vi "nanocal -- nuclear schottky fit V7.vi"() -> ()   [LabVIEW 2021] (continued)
\"T\" -> 0.830000000000   ,  \"B\" -> 0.000000000000   ,  \"θ\" -> 0.000000000000   ,  \"Reoff\" -> -3028571.428571429100   ,  \"Imoff\" -> 0.000000000000   ,  \"στ1\" -> 0.003777268036   ,  \"στS\" -> 0.001674973783   ,  \"στN\" -> 0.000298996570    |>   , \n\"IDS0417_220525_RAW_cal__sam_\" ->   <|    \"ζ\" -> 0.020422056832   ,  \"τ1\" -> 0.006457484957   ,  \"τS\" -> 0.019722165301   ,  \"τN\" -> 0.000729413719   ,  \"τC\" -> 0.001622930071   ,  \"κ0\" -> 0.000000005380   ,  \"mm1\" -> 0.000030097695   ,  \"mm2\" -> 0.006162713408   ,  \"mm3\" -> 0.022756846254   ,  \"T\" -> 0.830000000000   ,  \"B\" -> 0.000000000000   ,  \"θ\" -> 0.000000000000   ,  \"Reoff\" -> -2081632.653061224150   ,  \"Imoff\" -> 0.000000000000   ,  \"στ1\" -> 0.000977899540   ,  \"στS\" -> 0.002370947727   ,  \"στN\" -> 0.000160479256    |>   , \n\"IDS0418_220525_RAW_cal__ref_\" ->   <|    \"ζ\" -> 0.022904137166   ,  \"τ1\" -> 0.004842430213   ,  \"τS\" -> 0.021231337399   ,  \"τN\" -> 0.000595878691   ,  \"τC\" -> 0.001701256533   ,  \"κ0\" -> 0.000000006850   ,  \"mm1\" -> 0.000035378969   ,  \"mm2\" -> 0.004689611444   ,  \"mm3\" -> 0.024145845974   ,  \"T\" -> 1.120000000000   ,  \"B\" -> 0.000000000000   ,  \"θ\" -> 0.000000000000   ,  \"Reoff\" -> -1314285.714285716420   ,  \"Imoff\" -> 0.000000000000   ,  \"στ1\" -> 0.000594455147   ,  \"στS\" -> 0.001847173468   ,  \"στN\" -> 0.000101337306    |>   , \n\"IDS0418_220525_RAW_cal__sam_\" ->   <|    \"ζ\" -> 0.010833914814   ,  \"τ1\" -> 0.006105280968   ,  \"τS\" -> 0.027771405990   ,  \"τN\" -> 0.000655710517   ,  \"τC\" -> 0.001898693697   ,  \"κ0\" -> 0.000000007420   ,  \"mm1\" -> 0.000019072683   ,  \"mm2\" -> 0.005941306089   ,  \"mm3\" -> 0.030778689359   ,  \"T\" -> 1.120000000000   ,  \"B\" -> 0.000000000000   ,  \"θ\" -> 0.000000000000   ,  \"Reoff\" -> -608163.265306122367   ,  \"Imoff\" -> 0.000000000000   ,  \"στ1\" -> 0.001326459237   ,  \"στS\" -> 0.003728359065   ,  \"στN\" -> 0.000181682896    |>   , \n\"IDS0419_220525_RAW_cal__ref_\" ->   <|    \"ζ\" -> 0.019588015905   ,  \"τ1\" -> 0.004781626559   ,  \"τS\" -> 0.047742438651   ,  \"τN\" -> 0.000600848305   ,  \"τC\" -> 0.002316865749   ,  \"κ0\" -> 0.000000012200   ,  \"mm1\" -> 0.000042523875   ,  \"mm2\" -> 0.004719121437   ,  \"mm3\" -> 0.051627083026   ,  \"T\" -> 1.900000000000   ,  \"B\" -> 0.000000000000   ,  \"θ\" -> 0.000000000000   ,  \"Reoff\" -> -714285.714285716413   ,  \"Imoff\" -> 0.000000000000   ,  \"στ1\" -> 0.001059318885   ,  \"στS\" -> 0.005613918235   ,  \"στN\" -> 0.000174681152    |>   , \n\"IDS0419_220525_RAW_cal__sam_\" ->   <|    \"ζ\" -> 0.011595776290   ,  \"τ1\" -> 0.006117918264   ,  \"τS\" -> 0.061916055974   ,  \"τN\" -> 0.000669101537   ,  \"τC\" -> 0.002022450323   ,  \"κ0\" -> 0.000000012950   ,  \"mm1\" -> 0.000022465670   ,  \"mm2\" -> 0.006048051710   ,  \"mm3\" -> 0.065380732203   ,  \"T\" -> 1.900000000000   ,  \"B\" -> 0.000000000000   ,  \"θ\" -> 0.000000000000   ,  \"Reoff\" -> -608163.265306122367   ,  \"Imoff\" -> 0.000000000000   ,  \"στ1\" -> 0.001547930555   ,  \"στS\" -> 0.007827805463   ,  \"στN\" -> 0.000227173092    |>   , \n\"IDS0420_220525_RAW_cal__ref_\" ->   <|    \"ζ\" -> 0.020834428044   ,  \"τ1\" -> 0.004699063518   ,  \"τS\" -> 0.052089260804   ,  \"τN\" -> 0.000594934592   ,  \"τC\" -> 0.002174562230   ,  \"κ0\" -> 0.000000013800   ,  \"mm1\" -> 0.000042670178   ,  \"mm2\" -> 0.004643420551   ,  \"mm3\" -> 0.055969375493   ,  \"T\" -> 2.100000000000   ,  \"B\" -> 0.000000000000   ,  \"θ\" -> 0.000000000000   ,  \"Reoff\" -> -714285.714285716413   ,  \"Imoff\" -> 0.000000000000   ,  \"στ1\" -> 0.001320131062   ,  \"στS\" -> 0.004774189877   ,  \"στN\" -> 0.000170930701    |>   , \n\"IDS0420_220525_RAW_cal__sam_\" ->   <|    \"ζ\" -> 0.011850996022   ,  \"τ1\" -> 0.005764384736   ,  \"τS\" -> 0.066220067505   ,  \"τN\" -> 0.000645440877   ,  \"τC\" -> 0.002901198812   ,  \"κ0\" -> 0.000000014700   ,  \"mm1\" -> 0.000032584327   ,  \"mm2\" -> 0.005706320364   ,  \"mm3\" -> 0.070584610113   ,  \"T\" -> 2.100000000000   ,  \"B\" -> 0.000000000000   ,  \"θ\" -> 0.000000000000   ,  \"Reoff\" -> -461224.489795918343   ,  \"Imoff\" -> 0.000000000000   ,  \"στ1\" -> 0.000879947943   ,  \"στS\" -> 0.005816006372   ,  \"στN\" -> 0.000150645668    |>   , \n\"IDS0421_220525_RAW_cal__ref_\" ->   <|    \"ζ\" -> 0.022335092396   ,  \"τ1\" -> 0.004357676744   ,  \"τS\" -> 0.014734142286   ,  \"τN\" -> 0.000494755663   ,  \"τC\" -> 0.002291218216   ,  \"κ0\" -> 0.000000015200   ,  \"mm1\" -> 0.000043555244   ,  \"mm2\" -> 0.004196096690   ,  \"mm3\" -> 0.017978279817   ,  \"T\" -> 2.300000000000   ,  \"B\" -> 0.000000000000   ,  \"θ\" -> 0.000000000000   ,  \"Reoff\" -> -714285.714285716413   ,  \"Imoff\" -> 0.000000000000   ,  \"στ1\" -> 0.001017327919   ,  \"στS\" -> 0.002314643379   ,  \"στN\" -> 0.000146182526    |>   , \n\"IDS0421_220525_RAW_cal__sam_\" ->   <|    \"ζ\" -> 0.017472306497   ,  \"τ1\" -> 0.005884707777   ,  \"τS\" -> 0.018273540555   ,  \"τN\" -> 0.000393530305   ,  \"τC\" -> 0.002873982576   ,  \"κ0\" -> 0.000000016000   ,  \"mm1\" -> 0.000042829990   ,  \"mm2\" -> 0.005738391469   ,  \"mm3\" -> 0.021970696537   ,  \"T\" -> 2.300000000000   ,  \"B\" -> 0.000000000000   ,  \"θ\" -> 0.000000000000   ,  \"Reoff\" -> -616326.530612244968   ,  \"Imoff\" -> 0.000000000000   ,  \"στ1\" -> 0.001449504442   ,  \"στS\" -> 0.003094967894   ,  \"στN\" -> 0.000132016087    |>   , \n\"IDS0422_220525_RAW_cal__ref_\" ->   <|    \"ζ\" -> 0.018555902016   ,  \"τ1\" -> 0.004075291246   ,  \"τS\" -> 0.009145270052   ,  \"τN\" -> 0.000208864759   ,  \"τC\" -> 0.002022167505   ,  \"κ0\" -> 0.000000022500   ,  \"mm1\" -> 0.000030348931   ,  \"mm2\" -> 0.003960776557   ,  \"mm3\" -> 0.011634042483   ,  \"T\" -> 3.100000000000   ,  \"B\" -> 0.000000000000   ,  \"θ\" -> 0.000000000000   ,  \"Reoff\" -> -371428.571428570896   ,  \"Imoff\" -> 0.000000000000   ,  \"στ1\" -> 0.000657121780   ,  \"στS\" -> 0.001216403398   ,  \"στN\" -> 0.000050486757    |>   , \n\"IDS0422_220525_RAW_cal__sam_\" ->   <|    \"ζ\" -> 0.013782660001   ,  \"τ1\" -> 0.005602489845   ,  \"τS\" -> 0.011122141420   ,  \"τN\" -> 0.000341635093   ,  \"τC\" -> 0.002887063483   ,  \"κ0\" -> 0.000000023500   ,  \"mm1\" -> 0.000031317292   ,  \"mm2\" -> 0.005389288482   ,  \"mm3\" -> 0.014690725401   ,  \"T\" -> 3.100000000000   ,  \"B\" -> 0.000000000000   ,  \"θ\" -> 0.000000000000   ,  \"Reoff\" -> -338775.510204081656   ,  \"Imoff\" -> 0.000000000000   ,  \"στ1\" -> 0.000787586702   ,  \"στS\" -> 0.001319427978   ,  \"στN\" -> 0.000072408344    |>   , \n\"IDS0424_220526_RAW_cal__ref_\" ->   <|    \"ζ\" -> 0.257865003377   ,  \"τ1\" -> 0.052975439100   ,  \"τS\" -> 0.072879585760   ,  \"τN\" -> 0.046129702285   ,  \"τC\" -> 0.000850997737   ,  \"κ0\" -> 0.000000000770   ,  \"mm1\" -> 0.000173173247   ,  \"mm2\" -> 0.027881728109   ,  \"mm3\" -> 0.175469153990   ,  \"T\" -> 0.190000000000   ,  \"B\" -> 10.000000000000   ,  \"θ\" -> 0.000000000000   ,  \"Reoff\" -> -49000000.000000000000   ,  \"Imoff\" -> 0.000000000000   ,  \"στ1\" -> 0.038419382366   ,  \"στS\" -> 0.010252018344   ,  \"στN\" -> 0.015460977129    |>   , \n\"IDS0424_220526_RAW_cal__sam_\" ->   <|    \"ζ\" -> 0.143096873941   ,  \"τ1\" -> 0.119527741552   ,  \"τS\" -> 0.213771204505   ,  \"τN\" -> 0.133065206622   ,  \"τC\" -> 0.001041786526   ,  \"κ0\" -> 0.000000000890   ,  \"mm1\" -> 0.000129929317   ,  \"mm2\" -> 0.064852834373   ,  \"mm3\" -> 0.452054381716   ,  \"T\" -> 0.190000000000   ,  \"B\" -> 10.000000000000   ,  \"θ\" -> 0.000000000000   ,  \"Reoff\" -> -41461224.489795915800   ,  \"Imoff\" -> 0.000000000000   ,  \"στ1\" -> 0.142328196867   ,  \"στS\" -> 0.153709890516   ,  \"στN\" -> 0.034979737706    |>   , \n\"IDS0425_220526_RAW_cal__ref_\" ->   <|    \"ζ\" -> 0.150640974704   ,  \"τ1\" -> 0.034197272609   ,  \"τS\" -> 0.049670713863   ,  \"τN\" -> 0.019296596370   ,  \"τC\" -> 0.000986151726   ,  \"κ0\" -> 0.000000001118   ,  \"mm1\" -> 0.000127191823   ,  \"mm2\" -> 0.021308290346   ,  \"mm3\" -> 0.093104555235   ,  \"T\" -> 0.250000000000   ,  \"B\" -> 10.000000000000   ,  \"θ\" -> 0.000000000000   ,  \"Reoff\" -> -20330612.244897961600   ,  \"Imoff\" -> 0.000000000000   ,  \"στ1\" -> 0.016426599332   ,  \"στS\" -> 0.002938321228   ,  \"στN\" -> 0.003825151273    |>   , \n\"IDS0425_220526_RAW_cal__sam_\" ->   <|    \"ζ\" -> 0.080613368975   ,  \"τ1\" -> 0.039981630615   ,  \"τS\" -> 0.067451052819   ,  \"τN\" -> 0.024952731947   ,  \"τC\" -> 0.001301901326   ,  \"κ0\" -> 0.000000001270   ,  \"mm1\" -> 0.000095538727   ,  \"mm2\" -> 0.025680137218   ,  \"mm3\" -> 0.115360621158   ,  \"T\" -> 0.250000000000   ,  \"B\" -> 10.000000000000   ,  \"θ\" -> 0.000000000000   ,  \"Reoff\" -> -15077551.020408168400   ,  \"Imoff\" -> 0.000000000000   ,  \"στ1\" -> 0.017921325903   ,  \"στS\" -> 0.008554959302   ,  \"στN\" -> 0.012696106226    |>   , \n\"IDS0426_220526_RAW_cal__ref_\" ->   <|    \"ζ\" -> 0.110651122840   ,  \"τ1\" -> 0.023688979566   ,  \"τS\" -> 0.041888104291   ,  \"τN\" -> 0.009400965947   ,  \"τC\" -> 0.001054144270   ,  \"κ0\" -> 0.000000001430   ,  \"mm1\" -> 0.000102915193   ,  \"mm2\" -> 0.017560405745   ,  \"mm3\" -> 0.064044066348   ,  \"T\" -> 0.300000000000   ,  \"B\" -> 10.000000000000   ,  \"θ\" -> 0.000000000000   ,  \"Reoff\" -> -13408163.265306122600   ,  \"Imoff\" -> 0.000000000000   ,  \"στ1\" -> 0.009988334429   ,  \"στS\" -> 0.001537868285   ,  \"στN\" -> 0.001719296338    |>   , \n\"IDS0426_220526_RAW_cal__sam_\" ->   <|    \"ζ\" -> 0.000000000000   ,  \"τ1\" -> 0.000000000000   ,  \"τS\" -> 0.000000000000   ,  \"τN\" -> 0.000000000000   ,  \"τC\" -> 0.000000000000   ,  \"κ0\" -> 0.000000000000   ,  \"mm1\" -> 0.000000000000   ,  \"mm2\" -> 0.000000000000   ,  \"mm3\" -> 0.000000000000   ,  \"T\" -> 0.300000000000   ,  \"B\" -> 10.000000000000   ,  \"θ\" -> 0.000000000000   ,  \"Reoff\" -> 0.000000000000   ,  \"Imoff\" -> 0.000000000000   ,  \"στ1\" -> 0.000000000000   ,  \"στS\" -> 0.000000000000   ,  \"στN\" -> 0.000000000000    |>   , \n\"IDS0427_220526_RAW_cal__ref_\" ->   <|    \"ζ\" -> 0.400378368532   ,  \"τ1\" -> 0.070020543839   ,  \"τS\" -> 0.131128875469   ,  \"τN\" -> 0.110503953528   ,  \"τC\" -> 0.000929381263   ,  \"κ0\" -> 0.000000000547   ,  \"mm1\" -> 0.000264755544   ,  \"mm2\" -> 0.034447529222   ,  \"mm3\" -> 0.374615027191   ,  \"T\" -> 0.150000000000   ,  \"B\" -> 10.000000000000   ,  \"θ\" -> 0.000000000000   ,  \"Reoff\" -> -90065306.122448980800   ,  \"Imoff\" -> 0.000000000000   ,  \"στ1\" -> 0.115545840550   ,  \"στS\" -> 0.062145974598   ,  \"στN\" -> 0.087083233243    |>   , \n\"IDS0427_220526_RAW_cal__sam_\" ->   <|    \"ζ\" -> 0.000000000000   ,  \"τ1\" -> 0.000000000000   ,  \"τS\" -> 0.000000000000   ,  \"τN\" -> 0.000000000000   ,  \"τC\" -> 0.000000000000   ,  \"κ0\" -> 0.000000000000   ,  \"mm1\" -> 0.000000000000   ,  \"mm2\" -> 0.000000000000   ,  \"mm3\" -> 0.000000000000   ,  \"T\" -> 0.150000000000   ,  \"B\" -> 10.000000000000   ,  \"θ\" -> 0.000000000000   ,  \"Reoff\" -> 0.000000000000   ,  \"Imoff\" -> 0.000000000000   ,  \"στ1\" -> 0.000000000000   ,  \"στS\" -> 0.000000000000   ,  \"στN\" -> 0.000000000000    |>   , \n\"IDS0428_220526_RAW_cal__ref_\" ->   <|    \"ζ\" -> 0.082438962756   ,  \"τ1\" -> 0.024345135189   ,  \"τS\" -> 0.039010983719   ,  \"τN\" -> 0.005604008996   ,  \"τC\" -> 0.001011795266   ,  \"κ0\" -> 0.000000001850   ,  \"mm1\" -> 0.000075386231   ,  \"mm2\" -> 0.019395489677   ,  \"mm3\" -> 0.054179060985   ,  \"T\" -> 0.360000000000   ,  \"B\" -> 10.000000000000   ,  \"θ\" -> 0.000000000000   ,  \"Reoff\" -> -9632653.061224490410   ,  \"Imoff\" -> 0.000000000000   ,  \"στ1\" -> 0.001903743103   ,  \"στS\" -> 0.000574153374   ,  \"στN\" -> 0.002568840036    |>   , \n\"IDS0428_220526_RAW_cal__sam_\" ->   <|    \"ζ\" -> 0.000000000000   ,  \"τ1\" -> 0.000000000000   ,  \"τS\" -> 0.000000000000   ,  \"τN\" -> 0.000000000000   ,  \"τC\" -> 0.000000000000   ,  \"κ0\" -> 0.000000000000   ,  \"mm1\" -> 0.000000000000   ,  \"mm2\" -> 0.000000000000   ,  \"mm3\" -> 0.000000000000   ,  \"T\" -> 0.360000000000   ,  \"B\" -> 10.000000000000   ,  \"θ\" -> 0.000000000000   ,  \"Reoff\" -> 0.000000000000   ,  \"Imoff\" -> 0.000000000000   ,  \"στ1\" -> 0.000000000000   ,  \"στS\" -> 0.000000000000   ,  \"στN\" -> 0.000000000000    |>   , \n\"IDS0429_220526_RAW_cal__ref_\" ->   <|    \"ζ\" -> 0.070312011413   ,  \"τ1\" -> 0.022685637424   ,  \"τS\" -> 0.038017817435   ,  \"τN\" -> 0.003686111033   ,  \"τC\" -> 0.000858092615   ,  \"κ0\" -> 0.000000002230   ,  \"mm1\" -> 0.000055279779   ,  \"mm2\" -> 0.019266175315   ,  \"mm3\" -> 0.048858490507   ,  \"T\" -> 0.420000000000   ,  \"B\" -> 10.000000000000   ,  \"θ\" -> 0.000000000000   ,  \"Reoff\" -> -9632653.061224490410   ,  \"Imoff\" -> 0.000000000000   ,  \"στ1\" -> 0.001355990341   ,  \"στS\" -> 0.000271524957   ,  \"στN\" -> 0.000140246830    |>   , \n\"IDS0429_220526_RAW_cal__sam_\" ->   <|    \"ζ\" -> 0.000000000000   ,  \"τ1\" -> 0.000000000000   ,  \"τS\" -> 0.000000000000   ,  \"τN\" -> 0.000000000000   ,  \"τC\" -> 0.000000000000   ,  \"κ0\" -> 0.000000000000   ,  \"mm1\" -> 0.000000000000   ,  \"mm2\" -> 0.000000000000   ,  \"mm3\" -> 0.000000000000   ,  \"T\" -> 0.420000000000   ,  \"B\" -> 10.000000000000   ,  \"θ\" -> 0.000000000000   ,  \"Reoff\" -> 0.000000000000   ,  \"Imoff\" -> 0.000000000000   ,  \"στ1\" -> 0.000000000000   ,  \"στS\" -> 0.000000000000   ,  \"στN\" -> 0.000000000000    |>   , \n\"IDS0430_220526_RAW_cal__ref_\" ->   <|    \"ζ\" -> 0.045461152604   ,  \"τ1\" -> 0.022205538452   ,  \"τS\" -> 0.038393095410   ,  \"τN\" -> 0.002129809404   ,  \"τC\" -> 0.001500655488   ,  \"κ0\" -> 0.000000002910   ,  \"mm1\" -> 0.000062998174   ,  \"mm2\" -> 0.020118168551   ,  \"mm3\" -> 0.045890149989   ,  \"T\" -> 0.520000000000   ,  \"B\" -> 10.000000000000   ,  \"θ\" -> 0.000000000000   ,  \"Reoff\" -> -3224489.795918375260   ,  \"Imoff\" -> 0.000000000000   ,  \"στ1\" -> 0.001544196925   ,  \"στS\" -> 0.000197668706   ,  \"στN\" -> 0.000070756968    |>   , \n\"IDS0430_220526_RAW_cal__sam_\" ->   <|    \"ζ\" -> 0.000000000000   ,  \"τ1\" -> 0.000000000000   ,  \"τS\" -> 0.000000000000   ,  \"τN\" -> 0.000000000000   ,  \"τC\" -> 0.000000000000   ,  \"κ0\" -> 0.000000000000   ,  \"mm1\" -> 0.000000000000   ,  \"mm2\" -> 0.000000000000   ,  \"mm3\" -> 0.000000000000   ,  \"T\" -> 0.520000000000   ,  \"B\" -> 10.000000000000   ,  \"θ\" -> 0.000000000000   ,  \"Reoff\" -> 0.000000000000   ,  \"Imoff\" -> 0.000000000000   ,  \"στ1\" -> 0.000000000000   ,  \"στS\" -> 0.000000000000   ,  \"στN\" -> 0.000000000000    |>   , \n\"IDS0431_220527_RAW_cal__ref_\" ->   <|    \"ζ\" -> 0.560959524386   ,  \"τ1\" -> 0.162135875123   ,  \"τS\" -> 0.311559023690   ,  \"τN\" -> 0.235565493895   ,  \"τC\" -> 0.000943331482   ,  \"κ0\" -> 0.000000000415   ,  \"mm1\" -> 0.000338581832   ,  \"mm2\" -> 0.084703245290   ,  \"mm3\" -> 0.932076606233   ,  \"T\" -> 0.120000000000   ,  \"B\" -> 10.000000000000   ,  \"θ\" -> 0.000000000000   ,  \"Reoff\" -> -130387755.102040812000   ,  \"Imoff\" -> 0.000000000000   ,  \"στ1\" -> 0.196821258023   ,  \"στS\" -> 0.124985342591   ,  \"στN\" -> 0.122755892139    |>   , \n\"IDS0431_220527_RAW_cal__sam_\" ->   <|    \"ζ\" -> 0.000000000000   ,  \"τ1\" -> 0.000000000000   ,  \"τS\" -> 0.000000000000   ,  \"τN\" -> 0.000000000000   ,  \"τC\" -> 0.000000000000   ,  \"κ0\" -> 0.000000000000   ,  \"mm1\" -> 0.000000000000   ,  \"mm2\" -> 0.000000000000   ,  \"mm3\" -> 0.000000000000   ,  \"T\" -> 0.120000000000   ,  \"B\" -> 10.000000000000   ,  \"θ\" -> 0.000000000000   ,  \"Reoff\" -> 0.000000000000   ,  \"Imoff\" -> 0.000000000000   ,  \"στ1\" -> 0.000000000000   ,  \"στS\" -> 0.000000000000   ,  \"στN\" -> 0.000000000000    |>   , \n\"IDS0432_220527_RAW_cal__ref_\" ->   <|    \"ζ\" -> 0.302881771202   ,  \"τ1\" -> 0.053970650610   ,  \"τS\" -> 0.084832458604   ,  \"τN\" -> 0.070036651320   ,  \"τC\" -> 0.000864371133   ,  \"κ0\" -> 0.000000000675   ,  \"mm1\" -> 0.000199736141   ,  \"mm2\" -> 0.026051282095   ,  \"mm3\" -> 0.230360143749   ,  \"T\" -> 0.170000000000   ,  \"B\" -> 10.000000000000   ,  \"θ\" -> 0.000000000000   ,  \"Reoff\" -> -65714285.714285716400   ,  \"Imoff\" -> 0.000000000000   ,  \"στ1\" -> 0.042116863127   ,  \"στS\" -> 0.016985307293   ,  \"στN\" -> 0.023565277591    |>   , \n\"IDS0432_220527_RAW_cal__sam_\" ->   <|    \"ζ\" -> 0.000000000000   ,  \"τ1\" -> 0.000000000000   ,  \"τS\" -> 0.000000000000   ,  \"τN\" -> 0.000000000000   ,  \"τC\" -> 0.000000000000   ,  \"κ0\" -> 0.000000000000   ,  \"mm1\" -> 0.000000000000   ,  \"mm2\" -> 0.000000000000   ,  \"mm3\" -> 0.000000000000   ,  \"T\" -> 0.170000000000   ,  \"B\" -> 10.000000000000   ,  \"θ\" -> 0.000000000000   ,  \"Reoff\" -> 0.000000000000   ,  \"Imoff\" -> 0.000000000000   ,  \"στ1\" -> 0.000000000000   ,  \"στS\" -> 0.000000000000   ,  \"στN\" -> 0.000000000000    |>   , \n\"IDS0433_220527_RAW_cal__ref_\" ->   <|    \"ζ\" -> 0.035999178559   ,  \"τ1\" -> 0.021236822586   ,  \"τS\" -> 0.040779763241   ,  \"τN\" -> 0.001074221992   ,  \"τC\" -> 0.001739718615   ,  \"κ0\" -> 0.000000003576   ,  \"mm1\" -> 0.000058137989   ,  \"mm2\" -> 0.020282386509   ,  \"mm3\" -> 0.045996711024   ,  \"T\" -> 0.620000000000   ,  \"B\" -> 10.000000000000   ,  \"θ\" -> 0.000000000000   ,  \"Reoff\" -> -1959183.673469394450   ,  \"Imoff\" -> 0.000000000000   ,  \"στ1\" -> 0.001449693425   ,  \"στS\" -> 0.000173563135   ,  \"στN\" -> 0.000045450535    |>   , \n\"IDS0433_220527_RAW_cal__sam_\" ->   <|    \"ζ\" -> 0.000000000000   ,  \"τ1\" -> 0.000000000000   ,  \"τS\" -> 0.000000000000   ,  \"τN\" -> 0.000000000000   ,  \"τC\" -> 0.000000000000   ,  \"κ0\" -> 0.000000000000   ,  \"mm1\" -> 0.000000000000   ,  \"mm2\" -> 0.000000000000   ,  \"mm3\" -> 0.000000000000   ,  \"T\" -> 0.620000000000   ,  \"B\" -> 10.000000000000   ,  \"θ\" -> 0.000000000000   ,  \"Reoff\" -> 0.000000000000   ,  \"Imoff\" -> 0.000000000000   ,  \"στ1\" -> 0.000000000000   ,  \"στS\" -> 0.000000000000   ,  \"στN\" -> 0.000000000000    |>   , \n\"IDS0434_220527_RAW_cal__ref_\" ->   <|    \"ζ\" -> 0.027519355554   ,  \"τ1\" -> 0.020590521074   ,  \"τS\" -> 0.048137141101   ,  \"τN\" -> 0.000693113139   ,  \"τC\" -> 0.001789335146   ,  \"κ0\" -> 0.000000004950   ,  \"mm1\" -> 0.000046291190   ,  \"mm2\" -> 0.020129239579   ,  \"mm3\" -> 0.052378356819   ,  \"T\" -> 0.820000000000   ,  \"B\" -> 10.000000000000   ,  \"θ\" -> 0.000000000000   ,  \"Reoff\" -> -1326530.612244904040   ,  \"Imoff\" -> 0.000000000000   ,  \"στ1\" -> 0.000620759114   ,  \"στS\" -> 0.000219619310   ,  \"στN\" -> 0.000010903062    |>   , \n\"IDS0434_220527_RAW_cal__sam_\" ->   <|    \"ζ\" -> 0.000000000000   ,  \"τ1\" -> 0.000000000000   ,  \"τS\" -> 0.000000000000   ,  \"τN\" -> 0.000000000000   ,  \"τC\" -> 0.000000000000   ,  \"κ0\" -> 0.000000000000   ,  \"mm1\" -> 0.000000000000   ,  \"mm2\" -> 0.000000000000   ,  \"mm3\" -> 0.000000000000   ,  \"T\" -> 0.820000000000   ,  \"B\" -> 10.000000000000   ,  \"θ\" -> 0.000000000000   ,  \"Reoff\" -> 0.000000000000   ,  \"Imoff\" -> 0.000000000000   ,  \"στ1\" -> 0.000000000000   ,  \"στS\" -> 0.000000000000   ,  \"στN\" -> 0.000000000000    |>   , \n\"IDS0435_220527_RAW_cal__ref_\" ->   <|    \"ζ\" -> 0.020842861739   ,  \"τ1\" -> 0.020135384195   ,  \"τS\" -> 0.018612634604   ,  \"τN\" -> 0.000305402785   ,  \"τC\" -> 0.002204389625   ,  \"κ0\" -> 0.000000007040   ,  \"mm1\" -> 0.000040405722   ,  \"mm2\" -> 0.018212466466   ,  \"mm3\" -> 0.023399245059   ,  \"T\" -> 1.120000000000   ,  \"B\" -> 10.000000000000   ,  \"θ\" -> 0.000000000000   ,  \"Reoff\" -> -693877.551020413636   ,  \"Imoff\" -> 0.000000000000   ,  \"στ1\" -> 0.001444867016   ,  \"στS\" -> 0.000117188914   ,  \"στN\" -> 0.000006503631    |>   , \n\"IDS0435_220527_RAW_cal__sam_\" ->   <|    \"ζ\" -> 0.000000000000   ,  \"τ1\" -> 0.000000000000   ,  \"τS\" -> 0.000000000000   ,  \"τN\" -> 0.000000000000   ,  \"τC\" -> 0.000000000000   ,  \"κ0\" -> 0.000000000000   ,  \"mm1\" -> 0.000000000000   ,  \"mm2\" -> 0.000000000000   ,  \"mm3\" -> 0.000000000000   ,  \"T\" -> 1.120000000000   ,  \"B\" -> 10.000000000000   ,  \"θ\" -> 0.000000000000   ,  \"Reoff\" -> 0.000000000000   ,  \"Imoff\" -> 0.000000000000   ,  \"στ1\" -> 0.000000000000   ,  \"στS\" -> 0.000000000000   ,  \"στN\" -> 0.000000000000    |>   , \n\"IDS0436_220527_RAW_cal__ref_\" ->   <|    \"ζ\" -> 0.020634042480   ,  \"τ1\" -> 0.020416898580   ,  \"τS\" -> 0.013006754143   ,  \"τN\" -> 0.000157221748   ,  \"τC\" -> 0.001868338850   ,  \"κ0\" -> 0.000000012250   ,  \"mm1\" -> 0.000033184482   ,  \"mm2\" -> 0.014698009084   ,  \"mm3\" -> 0.020989645793   ,  \"T\" -> 1.900000000000   ,  \"B\" -> 10.000000000000   ,  \"θ\" -> 0.000000000000   ,  \"Reoff\" -> -693877.551020413636   ,  \"Imoff\" -> 0.000000000000   ,  \"στ1\" -> 0.001009802597   ,  \"στS\" -> 0.000108538250   ,  \"στN\" -> 0.000005592624    |>   , \n\"IDS0436_220527_RAW_cal__sam_\" ->   <|    \"ζ\" -> 0.000000000000   ,  \"τ1\" -> 0.000000000000   ,  \"τS\" -> 0.000000000000   ,  \"τN\" -> 0.000000000000   ,  \"τC\" -> 0.000000000000   ,  \"κ0\" -> 0.000000000000   ,  \"mm1\" -> 0.000000000000   ,  \"mm2\" -> 0.000000000000   ,  \"mm3\" -> 0.000000000000   ,  \"T\" -> 1.900000000000   ,  \"B\" -> 10.000000000000   ,  \"θ\" -> 0.000000000000   ,  \"Reoff\" -> 0.000000000000   ,  \"Imoff\" -> 0.000000000000   ,  \"στ1\" -> 0.000000000000   ,  \"στS\" -> 0.000000000000   ,  \"στN\" -> 0.000000000000    |>   , \n\"IDS0437_220527_RAW_cal__ref_\" ->   <|    \"ζ\" -> 0.017700486500   ,  \"τ1\" -> 0.021195716861   ,  \"τS\" -> 0.009553240691   ,  \"τN\" -> 0.000096318625   ,  \"τC\" -> 0.001777778444   ,  \"κ0\" -> 0.000000022000   ,  \"mm1\" -> 0.000026199986   ,  \"mm2\" -> 0.011360732885   ,  \"mm3\" -> 0.021406923644   ,  \"T\" -> 3.100000000000   ,  \"B\" -> 10.000000000000   ,  \"θ\" -> 0.000000000000   ,  \"Reoff\" -> -326530.612244898453   ,  \"Imoff\" -> 0.000000000000   ,  \"στ1\" -> 0.003823035587   ,  \"στS\" -> 0.000080670014   ,  \"στN\" -> 0.000008312416    |>   , \n\"IDS0437_220527_RAW_cal__sam_\" ->   <|    \"ζ\" -> 0.000000000000   ,  \"τ1\" -> 0.000000000000   ,  \"τS\" -> 0.000000000000   ,  \"τN\" -> 0.000000000000   ,  \"τC\" -> 0.000000000000   ,  \"κ0\" -> 0.000000000000   ,  \"mm1\" -> 0.000000000000   ,  \"mm2\" -> 0.000000000000   ,  \"mm3\" -> 0.000000000000   ,  \"T\" -> 3.100000000000   ,  \"B\" -> 10.000000000000   ,  \"θ\" -> 0.000000000000   ,  \"Reoff\" -> 0.000000000000   ,  \"Imoff\" -> 0.000000000000   ,  \"στ1\" -> 0.000000000000   ,  \"στS\" -> 0.000000000000   ,  \"στN\" -> 0.000000000000    |>   , \n\"IDS0438_220527_RAW_cal__ref_\" ->   <|    \"ζ\" -> 0.017333863476   ,  \"τ1\" -> 0.021487771905   ,  \"τS\" -> 0.006060943357   ,  \"τN\" -> 0.000094743973   ,  \"τC\" -> 0.001680463551   ,  \"κ0\" -> 0.000000054800   ,  \"mm1\" -> 0.000022565233   ,  \"mm2\" -> 0.007769356044   ,  \"mm3\" -> 0.021638703353   ,  \"T\" -> 5.700000000000   ,  \"B\" -> 10.000000000000   ,  \"θ\" -> 0.000000000000   ,  \"Reoff\" -> -102040.816326530650   ,  \"Imoff\" -> 0.000000000000   ,  \"στ1\" -> 0.003634760564   ,  \"στS\" -> 0.000066823566   ,  \"στN\" -> 0.000004946508    |>   , \n\"IDS0438_220527_RAW_cal__sam_\" ->   <|    \"ζ\" -> 0.000000000000   ,  \"τ1\" -> 0.000000000000   ,  \"τS\" -> 0.000000000000   ,  \"τN\" -> 0.000000000000   ,  \"τC\" -> 0.000000000000   ,  \"κ0\" -> 0.000000000000   ,  \"mm1\" -> 0.000000000000   ,  \"mm2\" -> 0.000000000000   ,  \"mm3\" -> 0.000000000000   ,  \"T\" -> 5.700000000000   ,  \"B\" -> 10.000000000000   ,  \"θ\" -> 0.000000000000   ,  \"Reoff\" -> 0.000000000000   ,  \"Imoff\" -> 0.000000000000   ,  \"στ1\" -> 0.000000000000   ,  \"στS\" -> 0.000000000000   ,  \"στN\" -> 0.000000000000    |>   , \n\"IDS0439_220527_RAW_cal__ref_\" ->   <|    \"ζ\" -> 0.020515660719   ,  \"τ1\" -> 0.020182411708   ,  \"τS\" -> 0.016419895032   ,  \"τN\" -> 0.000240616919   ,  \"τC\" -> 0.002259910162   ,  \"κ0\" -> 0.000000008010   ,  \"mm1\" -> 0.000040116981   ,  \"mm2\" -> 0.017425178232   ,  \"mm3\" -> 0.021979340018   ,  \"T\" -> 1.280000000000   ,  \"B\" -> 10.000000000000   ,  \"θ\" -> 0.000000000000   ,  \"Reoff\" -> -693877.551020413636   ,  \"Imoff\" -> 0.000000000000   ,  \"στ1\" -> 0.001720696083   ,  \"στS\" -> 0.000105898596   ,  \"στN\" -> 0.000011441558    |>   , \n\"IDS0439_220527_RAW_cal__sam_\" ->   <|    \"ζ\" -> 0.000000000000   ,  \"τ1\" -> 0.000000000000   ,  \"τS\" -> 0.000000000000   ,  \"τN\" -> 0.000000000000   ,  \"τC\" -> 0.000000000000   ,  \"κ0\" -> 0.000000000000   ,  \"mm1\" -> 0.000000000000   ,  \"mm2\" -> 0.000000000000   ,  \"mm3\" -> 0.000000000000   ,  \"T\" -> 1.280000000000   ,  \"B\" -> 10.000000000000   ,  \"θ\" -> 0.000000000000   ,  \"Reoff\" -> 0.000000000000   ,  \"Imoff\" -> 0.000000000000   ,  \"στ1\" -> 0.000000000000   ,  \"στS\" -> 0.000000000000   ,  \"στN\" -> 0.000000000000    |>   , \n\"IDS0441_220527_RAW_cal__ref_\" ->   <|    \"ζ\" -> 0.245298177404   ,  \"τ1\" -> 0.085385227960   ,  \"τS\" -> 0.023089892303   ,  \"τN\" -> 0.011485885148   ,  \"τC\" -> 0.000787848696   ,  \"κ0\" -> 0.000000000810   ,  \"mm1\" -> 0.000151828666   ,  \"mm2\" -> 0.023847632864   ,  \"mm3\" -> 0.105230767769   ,  \"T\" -> 0.200000000000   ,  \"B\" -> 6.000000000000   ,  \"θ\" -> 0.000000000000   ,  \"Reoff\" -> -50367346.938775539400   ,  \"Imoff\" -> 0.000000000000   ,  \"στ1\" -> 0.073805144246   ,  \"στS\" -> 0.000832804395   ,  \"στN\" -> 0.007851231526    |>   , \n\"IDS0441_220527_RAW_cal__sam_\" ->   <|    \"ζ\" -> 0.000000000000   ,  \"τ1\" -> 0.000000000000   ,  \"τS\" -> 0.000000000000   ,  \"τN\" -> 0.000000000000   ,  \"τC\" -> 0.000000000000   ,  \"κ0\" -> 0.000000000000   ,  \"mm1\" -> 0.000000000000   ,  \"mm2\" -> 0.000000000000   ,  \"mm3\" -> 0.000000000000   ,  \"T\" -> 0.200000000000   ,  \"B\" -> 6.000000000000   ,  \"θ\" -> 0.000000000000   ,  \"Reoff\" -> 0.000000000000   ,  \"Imoff\" -> 0.000000000000   ,  \"στ1\" -> 0.000000000000   ,  \"στS\" -> 0.000000000000   ,  \"στN\" -> 0.000000000000    |>   , \n\"IDS0442_220528_RAW_cal__ref_\" ->   <|    \"ζ\" -> 0.649253803207   ,  \"τ1\" -> 0.189967266824   ,  \"τS\" -> 0.078891800944   ,  \"τN\" -> 0.111026532234   ,  \"τC\" -> 0.000810885423   ,  \"κ0\" -> 0.000000000435   ,  \"mm1\" -> 0.000318009867   ,  \"mm2\" -> 0.055339104870   ,  \"mm3\" -> 0.448344570802   ,  \"T\" -> 0.120000000000   ,  \"B\" -> 6.000000000000   ,  \"θ\" -> 0.000000000000   ,  \"Reoff\" -> -187755102.040816367000   ,  \"Imoff\" -> 0.000000000000   ,  \"στ1\" -> 0.116072095960   ,  \"στS\" -> 0.013830964310   ,  \"στN\" -> 0.055132667771    |>   , \n\"IDS0442_220528_RAW_cal__sam_\" ->   <|    \"ζ\" -> 0.000000000000   ,  \"τ1\" -> 0.000000000000   ,  \"τS\" -> 0.000000000000   ,  \"τN\" -> 0.000000000000   ,  \"τC\" -> 0.000000000000   ,  \"κ0\" -> 0.000000000000   ,  \"mm1\" -> 0.000000000000   ,  \"mm2\" -> 0.000000000000   ,  \"mm3\" -> 0.000000000000   ,  \"T\" -> 0.120000000000   ,  \"B\" -> 6.000000000000   ,  \"θ\" -> 0.000000000000   ,  \"Reoff\" -> 0.000000000000   ,  \"Imoff\" -> 0.000000000000   ,  \"στ1\" -> 0.000000000000   ,  \"στS\" -> 0.000000000000   ,  \"στN\" -> 0.000000000000    |>   , \n\"IDS0443_220528_RAW_cal__ref_\" ->   <|    \"ζ\" -> 0.445042406972   ,  \"τ1\" -> 0.128589504516   ,  \"τS\" -> 0.034654563108   ,  \"τN\" -> 0.043810211880   ,  \"τC\" -> 0.000810309510   ,  \"κ0\" -> 0.000000000605   ,  \"mm1\" -> 0.000246774346   ,  \"mm2\" -> 0.030747670130   ,  \"mm3\" -> 0.211790296861   ,  \"T\" -> 0.150000000000   ,  \"B\" -> 6.000000000000   ,  \"θ\" -> 0.000000000000   ,  \"Reoff\" -> -104489795.918367386000   ,  \"Imoff\" -> 0.000000000000   ,  \"στ1\" -> 0.161783937181   ,  \"στS\" -> 0.005303891089   ,  \"στN\" -> 0.043224722423    |>   , \n\"IDS0443_220528_RAW_cal__sam_\" ->   <|    \"ζ\" -> 0.000000000000   ,  \"τ1\" -> 0.000000000000   ,  \"τS\" -> 0.000000000000   ,  \"τN\" -> 0.000000000000   ,  \"τC\" -> 0.000000000000   ,  \"κ0\" -> 0.000000000000   ,  \"mm1\" -> 0.000000000000   ,  \"mm2\" -> 0.000000000000   ,  \"mm3\" -> 0.000000000000   ,  \"T\" -> 0.150000000000   ,  \"B\" -> 6.000000000000   ,  \"θ\" -> 0.000000000000   ,  \"Reoff\" -> 0.000000000000   ,  \"Imoff\" -> 0.000000000000   ,  \"στ1\" -> 0.000000000000   ,  \"στS\" -> 0.000000000000   ,  \"στN\" -> 0.000000000000    |>   , \n\"IDS0444_220528_RAW_cal__ref_\" ->   <|    \"ζ\" -> 0.346175274834   ,  \"τ1\" -> 0.111956082957   ,  \"τS\" -> 0.027343356843   ,  \"τN\" -> 0.025121384600   ,  \"τC\" -> 0.000749531065   ,  \"κ0\" -> 0.000000000740   ,  \"mm1\" -> 0.000189854194   ,  \"mm2\" -> 0.026751880765   ,  \"mm3\" -> 0.156390616794   ,  \"T\" -> 0.170000000000   ,  \"B\" -> 6.000000000000   ,  \"θ\" -> 0.000000000000   ,  \"Reoff\" -> -71183673.469387769700   ,  \"Imoff\" -> 0.000000000000   ,  \"στ1\" -> 0.050375037721   ,  \"στS\" -> 0.001079416051   ,  \"στN\" -> 0.009083705323    |>   , \n\"IDS0444_220528_RAW_cal__sam_\" ->   <|    \"ζ\" -> 0.000000000000   ,  \"τ1\" -> 0.000000000000   ,  \"τS\" -> 0.000000000000   ,  \"τN\" -> 0.000000000000   ,  \"τC\" -> 0.000000000000   ,  \"κ0\" -> 0.000000000000   ,  \"mm1\" -> 0.000000000000   ,  \"mm2\" -> 0.000000000000   ,  \"mm3\" -> 0.000000000000   ,  \"T\" -> 0.170000000000   ,  \"B\" -> 6.000000000000   ,  \"θ\" -> 0.000000000000   ,  \"Reoff\" -> 0.000000000000   ,  \"Imoff\" -> 0.000000000000   ,  \"στ1\" -> 0.000000000000   ,  \"στS\" -> 0.000000000000   ,  \"στN\" -> 0.000000000000    |>   , \n\"IDS0445_220528_RAW_cal__ref_\" ->   <|    \"ζ\" -> 0.167396769386   ,  \"τ1\" -> 0.076975995678   ,  \"τS\" -> 0.019126902976   ,  \"τN\" -> 0.005930151482   ,  \"τC\" -> 0.000960075113   ,  \"κ0\" -> 0.000000001240   ,  \"mm1\" -> 0.000132747039   ,  \"mm2\" -> 0.020623110398   ,  \"mm3\" -> 0.086431737778   ,  \"T\" -> 0.250000000000   ,  \"B\" -> 6.000000000000   ,  \"θ\" -> 0.000000000000   ,  \"Reoff\" -> -21224489.795918405100   ,  \"Imoff\" -> 0.000000000000   ,  \"στ1\" -> 0.058389287380   ,  \"στS\" -> 0.000426789295   ,  \"στN\" -> 0.003784929464    |>   , \n\"IDS0445_220528_RAW_cal__sam_\" ->   <|    \"ζ\" -> 0.000000000000   ,  \"τ1\" -> 0.000000000000   ,  \"τS\" -> 0.000000000000   ,  \"τN\" -> 0.000000000000   ,  \"τC\" -> 0.000000000000   ,  \"κ0\" -> 0.000000000000   ,  \"mm1\" -> 0.000000000000   ,  \"mm2\" -> 0.000000000000   ,  \"mm3\" -> 0.000000000000   ,  \"T\" -> 0.250000000000   ,  \"B\" -> 6.000000000000   ,  \"θ\" -> 0.000000000000   ,  \"Reoff\" -> 0.000000000000   ,  \"Imoff\" -> 0.000000000000   ,  \"στ1\" -> 0.000000000000   ,  \"στS\" -> 0.000000000000   ,  \"στN\" -> 0.000000000000    |>   , \n\"IDS0446_220528_RAW_cal__ref_\" ->   <|    \"ζ\" -> 0.116182318026   ,  \"τ1\" -> 0.081640310959   ,  \"τS\" -> 0.017704747394   ,  \"τN\" -> 0.003731217958   ,  \"τC\" -> 0.001140395347   ,  \"κ0\" -> 0.000000001560   ,  \"mm1\" -> 0.000112833833   ,  \"mm2\" -> 0.019484161721   ,  \"mm3\" -> 0.087110156248   ,  \"T\" -> 0.300000000000   ,  \"B\" -> 6.000000000000   ,  \"θ\" -> 0.000000000000   ,  \"Reoff\" -> -9836734.693877555430   ,  \"Imoff\" -> 0.000000000000   ,  \"στ1\" -> 0.008773282825   ,  \"στS\" -> 0.000191111466   ,  \"στN\" -> 0.000539753002    |>   , \n\"IDS0446_220528_RAW_cal__sam_\" ->   <|    \"ζ\" -> 0.000000000000   ,  \"τ1\" -> 0.000000000000   ,  \"τS\" -> 0.000000000000   ,  \"τN\" -> 0.000000000000   ,  \"τC\" -> 0.000000000000   ,  \"κ0\" -> 0.000000000000   ,  \"mm1\" -> 0.000000000000   ,  \"mm2\" -> 0.000000000000   ,  \"mm3\" -> 0.000000000000   ,  \"T\" -> 0.300000000000   ,  \"B\" -> 6.000000000000   ,  \"θ\" -> 0.000000000000   ,  \"Reoff\" -> 0.000000000000   ,  \"Imoff\" -> 0.000000000000   ,  \"στ1\" -> 0.000000000000   ,  \"στS\" -> 0.000000000000   ,  \"στN\" -> 0.000000000000    |>   , \n\"IDS0447_220528_RAW_cal__ref_\" ->   <|    \"ζ\" -> 0.082260507955   ,  \"τ1\" -> 0.097855412168   ,  \"τS\" -> 0.016892570352   ,  \"τN\" -> 0.002508450839   ,  \"τC\" -> 0.001377537548   ,  \"κ0\" -> 0.000000001980   ,  \"mm1\" -> 0.000097853534   ,  \"mm2\" -> 0.018911725587   ,  \"mm3\" -> 0.101220329644   ,  \"T\" -> 0.360000000000   ,  \"B\" -> 6.000000000000   ,  \"θ\" -> 0.000000000000   ,  \"Reoff\" -> -5918367.346938773990   ,  \"Imoff\" -> 0.000000000000   ,  \"στ1\" -> 0.011453835747   ,  \"στS\" -> 0.000169259584   ,  \"στN\" -> 0.000081203504    |>   , \n\"IDS0447_220528_RAW_cal__sam_\" ->   <|    \"ζ\" -> 0.000000000000   ,  \"τ1\" -> 0.000000000000   ,  \"τS\" -> 0.000000000000   ,  \"τN\" -> 0.000000000000   ,  \"τC\" -> 0.000000000000   ,  \"κ0\" -> 0.000000000000   ,  \"mm1\" -> 0.000000000000   ,  \"mm2\" -> 0.000000000000   ,  \"mm3\" -> 0.000000000000   ,  \"T\" -> 0.360000000000   ,  \"B\" -> 6.000000000000   ,  \"θ\" -> 0.000000000000   ,  \"Reoff\" -> 0.000000000000   ,  \"Imoff\" -> 0.000000000000   ,  \"στ1\" -> 0.000000000000   ,  \"στS\" -> 0.000000000000   ,  \"στN\" -> 0.000000000000    |>   , \n\"IDS0448_220528_RAW_cal__ref_\" ->   <|    \"ζ\" -> 0.062921401678   ,  \"τ1\" -> 0.104858235464   ,  \"τS\" -> 0.016995205436   ,  \"τN\" -> 0.001995569768   ,  \"τC\" -> 0.001676394953   ,  \"κ0\" -> 0.000000002390   ,  \"mm1\" -> 0.000091230686   ,  \"mm2\" -> 0.019175235813   ,  \"mm3\" -> 0.107453865317   ,  \"T\" -> 0.420000000000   ,  \"B\" -> 6.000000000000   ,  \"θ\" -> 0.000000000000   ,  \"Reoff\" -> -3224489.795918367800   ,  \"Imoff\" -> 0.000000000000   ,  \"στ1\" -> 0.006534185660   ,  \"στS\" -> 0.000117840372   ,  \"στN\" -> 0.000044604880    |>   , \n\"IDS0448_220528_RAW_cal__sam_\" ->   <|    \"ζ\" -> 0.000000000000   ,  \"τ1\" -> 0.000000000000   ,  \"τS\" -> 0.000000000000   ,  \"τN\" -> 0.000000000000   ,  \"τC\" -> 0.000000000000   ,  \"κ0\" -> 0.000000000000   ,  \"mm1\" -> 0.000000000000   ,  \"mm2\" -> 0.000000000000   ,  \"mm3\" -> 0.000000000000   ,  \"T\" -> 0.420000000000   ,  \"B\" -> 6.000000000000   ,  \"θ\" -> 0.000000000000   ,  \"Reoff\" -> 0.000000000000   ,  \"Imoff\" -> 0.000000000000   ,  \"στ1\" -> 0.000000000000   ,  \"στS\" -> 0.000000000000   ,  \"στN\" -> 0.000000000000    |>   , \n\"IDS0449_220528_RAW_cal__ref_\" ->   <|    \"ζ\" -> 0.047884623717   ,  \"τ1\" -> 0.131080457695   ,  \"τS\" -> 0.018007411450   ,  \"τN\" -> 0.000981367223   ,  \"τC\" -> 0.001725529599   ,  \"κ0\" -> 0.000000003050   ,  \"mm1\" -> 0.000072499299   ,  \"mm2\" -> 0.020333963628   ,  \"mm3\" -> 0.132297573561   ,  \"T\" -> 0.520000000000   ,  \"B\" -> 6.000000000000   ,  \"θ\" -> 0.000000000000   ,  \"Reoff\" -> -2734693.877551019190   ,  \"Imoff\" -> 0.000000000000   ,  \"στ1\" -> 0.004608574933   ,  \"στS\" -> 0.000117579650   ,  \"στN\" -> 0.000012752595    |>   , \n\"IDS0449_220528_RAW_cal__sam_\" ->   <|    \"ζ\" -> 0.000000000000   ,  \"τ1\" -> 0.000000000000   ,  \"τS\" -> 0.000000000000   ,  \"τN\" -> 0.000000000000   ,  \"τC\" -> 0.000000000000   ,  \"κ0\" -> 0.000000000000   ,  \"mm1\" -> 0.000000000000   ,  \"mm2\" -> 0.000000000000   ,  \"mm3\" -> 0.000000000000   ,  \"T\" -> 0.520000000000   ,  \"B\" -> 6.000000000000   ,  \"θ\" -> 0.000000000000   ,  \"Reoff\" -> 0.000000000000   ,  \"Imoff\" -> 0.000000000000   ,  \"στ1\" -> 0.000000000000   ,  \"στS\" -> 0.000000000000   ,  \"στN\" -> 0.000000000000    |>   , \n\"IDS0450_220528_RAW_cal__ref_\" ->   <|    \"ζ\" -> 0.039229464810   ,  \"τ1\" -> 0.132250871958   ,  \"τS\" -> 0.019567524350   ,  \"τN\" -> 0.000645572028   ,  \"τC\" -> 0.002216107396   ,  \"κ0\" -> 0.000000003710   ,  \"mm1\" -> 0.000075688104   ,  \"mm2\" -> 0.022339257593   ,  \"mm3\" -> 0.133058078988   ,  \"T\" -> 0.620000000000   ,  \"B\" -> 6.000000000000   ,  \"θ\" -> 0.000000000000   ,  \"Reoff\" -> -1836734.693877549840   ,  \"Imoff\" -> 0.000000000000   ,  \"στ1\" -> 0.013891983729   ,  \"στS\" -> 0.000275228505   ,  \"στN\" -> 0.000014669309    |>   , \n\"IDS0450_220528_RAW_cal__sam_\" ->   <|    \"ζ\" -> 0.000000000000   ,  \"τ1\" -> 0.000000000000   ,  \"τS\" -> 0.000000000000   ,  \"τN\" -> 0.000000000000   ,  \"τC\" -> 0.000000000000   ,  \"κ0\" -> 0.000000000000   ,  \"mm1\" -> 0.000000000000   ,  \"mm2\" -> 0.000000000000   ,  \"mm3\" -> 0.000000000000   ,  \"T\" -> 0.620000000000   ,  \"B\" -> 6.000000000000   ,  \"θ\" -> 0.000000000000   ,  \"Reoff\" -> 0.000000000000   ,  \"Imoff\" -> 0.000000000000   ,  \"στ1\" -> 0.000000000000   ,  \"στS\" -> 0.000000000000   ,  \"στN\" -> 0.000000000000    |>   , \n\"IDS0451_220528_RAW_cal__ref_\" ->   <|    \"ζ\" -> 0.026807399567   ,  \"τ1\" -> 0.154252177981   ,  \"τS\" -> 0.023590031432   ,  \"τN\" -> 0.000319958180   ,  \"τC\" -> 0.003023021175   ,  \"κ0\" -> 0.000000005180   ,  \"mm1\" -> 0.000070348215   ,  \"mm2\" -> 0.027105077142   ,  \"mm3\" -> 0.154650728056   ,  \"T\" -> 0.820000000000   ,  \"B\" -> 6.000000000000   ,  \"θ\" -> 0.000000000000   ,  \"Reoff\" -> -612244.897959182038   ,  \"Imoff\" -> 0.000000000000   ,  \"στ1\" -> 0.012428803494   ,  \"στS\" -> 0.000182806750   ,  \"στN\" -> 0.000002712737    |>   , \n\"IDS0451_220528_RAW_cal__sam_\" ->   <|    \"ζ\" -> 0.000000000000   ,  \"τ1\" -> 0.000000000000   ,  \"τS\" -> 0.000000000000   ,  \"τN\" -> 0.000000000000   ,  \"τC\" -> 0.000000000000   ,  \"κ0\" -> 0.000000000000   ,  \"mm1\" -> 0.000000000000   ,  \"mm2\" -> 0.000000000000   ,  \"mm3\" -> 0.000000000000   ,  \"T\" -> 0.820000000000   ,  \"B\" -> 6.000000000000   ,  \"θ\" -> 0.000000000000   ,  \"Reoff\" -> 0.000000000000   ,  \"Imoff\" -> 0.000000000000   ,  \"στ1\" -> 0.000000000000   ,  \"στS\" -> 0.000000000000   ,  \"στN\" -> 0.000000000000    |>   , \n\"IDS0452_220528_RAW_cal__ref_\" ->   <|    \"ζ\" -> 0.022314359927   ,  \"τ1\" -> 0.160926117275   ,  \"τS\" -> 0.032134640679   ,  \"τN\" -> 0.000145739971   ,  \"τC\" -> 0.002824145065   ,  \"κ0\" -> 0.000000007200   ,  \"mm1\" -> 0.000056854280   ,  \"mm2\" -> 0.035576714114   ,  \"mm3\" -> 0.161117390629   ,  \"T\" -> 1.120000000000   ,  \"B\" -> 6.000000000000   ,  \"θ\" -> 0.000000000000   ,  \"Reoff\" -> -702040.816326530649   ,  \"Imoff\" -> 0.000000000000   ,  \"στ1\" -> 0.054678579319   ,  \"στS\" -> 0.000310139427   ,  \"στN\" -> 0.000011071963    |>   , \n\"IDS0452_220528_RAW_cal__sam_\" ->   <|    \"ζ\" -> 0.000000000000   ,  \"τ1\" -> 0.000000000000   ,  \"τS\" -> 0.000000000000   ,  \"τN\" -> 0.000000000000   ,  \"τC\" -> 0.000000000000   ,  \"κ0\" -> 0.000000000000   ,  \"mm1\" -> 0.000000000000   ,  \"mm2\" -> 0.000000000000   ,  \"mm3\" -> 0.000000000000   ,  \"T\" -> 1.120000000000   ,  \"B\" -> 6.000000000000   ,  \"θ\" -> 0.000000000000   ,  \"Reoff\" -> 0.000000000000   ,  \"Imoff\" -> 0.000000000000   ,  \"στ1\" -> 0.000000000000   ,  \"στS\" -> 0.000000000000   ,  \"στN\" -> 0.000000000000    |>   , \n\"IDS0453_220529_RAW_cal__ref_\" ->   <|    \"ζ\" -> 0.018679261222   ,  \"τ1\" -> 0.150357444962   ,  \"τS\" -> 0.034780809519   ,  \"τN\" -> 0.000073406760   ,  \"τC\" -> 0.002819029609   ,  \"κ0\" -> 0.000000011200   ,  \"mm1\" -> 0.000047942172   ,  \"mm2\" -> 0.038176131794   ,  \"mm3\" -> 0.150457667894   ,  \"T\" -> 1.700000000000   ,  \"B\" -> 6.000000000000   ,  \"θ\" -> 0.000000000000   ,  \"Reoff\" -> -297959.183673469349   ,  \"Imoff\" -> 0.000000000000   ,  \"στ1\" -> 0.025512305357   ,  \"στS\" -> 0.000555960803   ,  \"στN\" -> 0.000005395580    |>   , \n\"IDS0453_220529_RAW_cal__sam_\" ->   <|    \"ζ\" -> 0.000000000000   ,  \"τ1\" -> 0.000000000000   ,  \"τS\" -> 0.000000000000   ,  \"τN\" -> 0.000000000000   ,  \"τC\" -> 0.000000000000   ,  \"κ0\" -> 0.000000000000   ,  \"mm1\" -> 0.000000000000   ,  \"mm2\" -> 0.000000000000   ,  \"mm3\" -> 0.000000000000   ,  \"T\" -> 1.700000000000   ,  \"B\" -> 6.000000000000   ,  \"θ\" -> 0.000000000000   ,  \"Reoff\" -> 0.000000000000   ,  \"Imoff\" -> 0.000000000000   ,  \"στ1\" -> 0.000000000000   ,  \"στS\" -> 0.000000000000   ,  \"στN\" -> 0.000000000000    |>   , \n\"IDS0454_220529_RAW_cal__ref_\" ->   <|    \"ζ\" -> 0.017513842872   ,  \"τ1\" -> 0.023424290493   ,  \"τS\" -> 0.014683078864   ,  \"τN\" -> 
